vi "#197-Caller flow of async message.vi"() -> ()   [LabVIEW 2017]
uses:
  user.lib/_NEVSTOP/Communicable State Machine(CSM)/_Support/Priority Queue/Priority Queue.lvclass/Priority Queue.ctl
  user.lib/_NEVSTOP/Communicable State Machine(CSM)/Utility/Build Error Cluster.vi
  user.lib/_NEVSTOP/Communicable State Machine(CSM)/Utility/uuid.vi
  user.lib/_NEVSTOP/Communicable State Machine(CSM)/_Support/Process/CSMP-Async Call.vi
  user.lib/_NEVSTOP/Communicable State Machine(CSM)/Utility/Trim Both Whitespace.vi
  user.lib/_NEVSTOP/Communicable State Machine(CSM)/_Support/CSMQ/_CSMObj-Message Check.vi
  user.lib/_NEVSTOP/Communicable State Machine(CSM)/_Support/CSMQ/_CSMObj-Enqueue Cross-Module Message.vi
  user.lib/_NEVSTOP/Communicable State Machine(CSM)/_Support/CSMQ/_CSMOFGV Get.vi
  user.lib/_NEVSTOP/Communicable State Machine(CSM)/_Support/Priority Queue/Enqueue Element.vi
  user.lib/_NEVSTOP/Communicable State Machine(CSM)/_Support/CSMQ/_CSMOFGV.vi
  user.lib/_NEVSTOP/Communicable State Machine(CSM)/Communicable State Machine.lvlib
panel:
  out "#msg to be processed":i32
  out "Diff Timer(s)":dbl format="%.6f"
  out "error IO":errorcluster
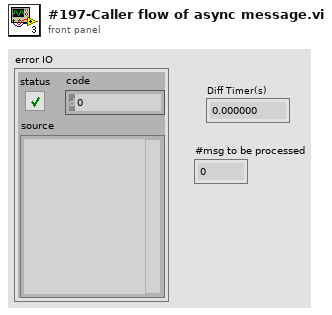
[diagram p1: front panel]
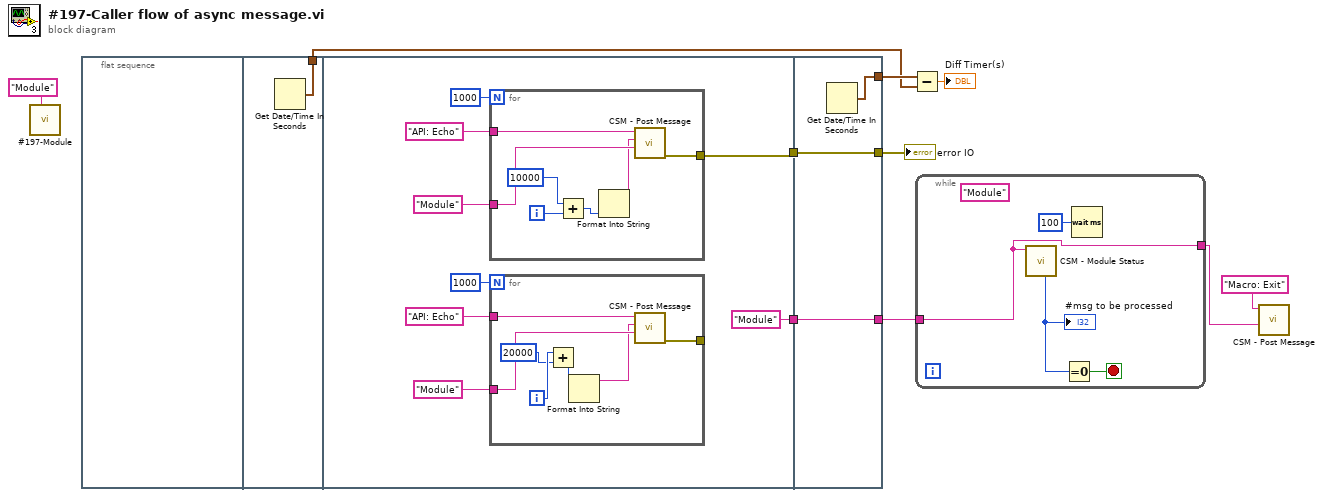
[diagram p0: block diagram]
diagram:
  n1 = call "#197-Module.vi"("Name(\"\" to use uuid)"="Module" ("Name(\"\" to use uuid)")) -> ()  [unwired: 11 in]
  n2 = flat-sequence {
    tunnel: [w11] -> w4
    tunnel: [w15] -> w8
    tunnel: ["Module" ("Name(\"\" to use uuid)")] -> w7
    tunnel: [w35] -> w2
    tunnel: [w36] -> w9
    tunnel: w8 -> [w36]
    tunnel: w7 -> [w35]
    tunnel: [w34] -> w6
    frame #0 {
    }
    frame #1 {
      n3 = Get Date/Time In Seconds() -> (seconds since 1Jan1904=w11:timestamp)
    }
    frame #2 {
      n4 = for {
        N: 1000 -> [_]
        tunnel: "API: Echo" ("State") -> [w33]
        tunnel: "Module" ("Name(\"\" to use uuid)") -> [w32]
        tunnel: [w31] -> w15
        i -> [w29]
        n5 = Add(x=10000, y=w29) -> (x+y=w28:i32)
        n6 = Format Into String(w28) -> (resulting string=w30:string)  [unwired: 3 in, 1 out]
        n7 = call "CSM - Post Message.vi"("Target Module"=w32, "Arguments (\"\")"=w30, "State"=w33) -> ("error out"=w31:errorcluster)  [unwired: 8 in]
      }
      n8 = for {
        N: 1000 -> [_]
        tunnel: "API: Echo" ("State") -> [w26]
        tunnel: "Module" ("Name(\"\" to use uuid)") -> [w25]
        tunnel: [w24] -> _
        i -> [w23]
        n9 = Add(x=w23, y=20000 ("x")) -> (x+y=w21:i32)
        n10 = Format Into String(w21) -> (resulting string=w22:string)  [unwired: 3 in, 1 out]
        n11 = call "CSM - Post Message.vi"("Target Module"=w25, "Arguments (\"\")"=w22, "State"=w26) -> ("error out"=w24:errorcluster)  [unwired: 8 in]
      }
    }
    frame #3 {
      n12 = Get Date/Time In Seconds() -> (seconds since 1Jan1904=w34:timestamp)
    }
  }
  n13 = Subtract(x=w6, y=w4) -> (x-y=→"Diff Timer(s)":dbl)
  n14 = while {
    tunnel: w2 -> [w37]
    tunnel: [w37] -> w1
    stop <- w39 stop-if-true
    (unwired) "Module" ("Name(\"\" to use uuid)")
    n15 = call "CSM - Module Status.vi"("CSM Name"=w37) -> ("#msg to be processed"=w40:i32)  [unwired: 6 in, 4 out]
    "#msg to be processed" <- w40
    n16 = Equal To 0?(x=w40) -> (x = 0?=w39:bool)
    n17 = Wait (ms)(milliseconds to wait=u32 100) -> ()  [unwired: 1 out]
  }
  n18 = call "CSM - Post Message.vi"("Target Module"=w1, "State"="Macro: Exit") -> ()  [unwired: 9 in, 1 out]
  "error IO" <- w9
